vi "Create Channels.vi"(8 "error in (no error)":errorcluster, 10 "RSI Module in":refnum<class "9401.lvclass">, 11 "Parent Ref in":T1 format="%.0x") -> (0 "error out":errorcluster, 2 "RSI Module out":refnum<class "9401.lvclass">, 3 "Parent Ref out":T1 format="%.0x")   [LabVIEW 2017, in "Modules.lvlib" / "9401.lvclass"]
uses:
  9401.lvclass
  C:/Users/dbuck/Documents/GitHub/Scan-Engine-Custom-Device-Classes/Source/RSI Module/RSI Module.lvclass
  <vilib>/NI Veristand/Custom Device API/Custom Device Item Ref.ctl
  <vilib>/NI Veristand/Custom Device API/Custom Device Channel Type.ctl
  <vilib>/NI Veristand/Custom Device API/Custom Device Channel.ctl
  9401.lvclass/9401.ctl
  RSI Module/Class Property Strings.vi
  RSI Module/Channel GUIDs.vi
  <vilib>/NI Veristand/Custom Device API/Custom Device API.lvlib
  RSI Module/RSI Module.lvclass
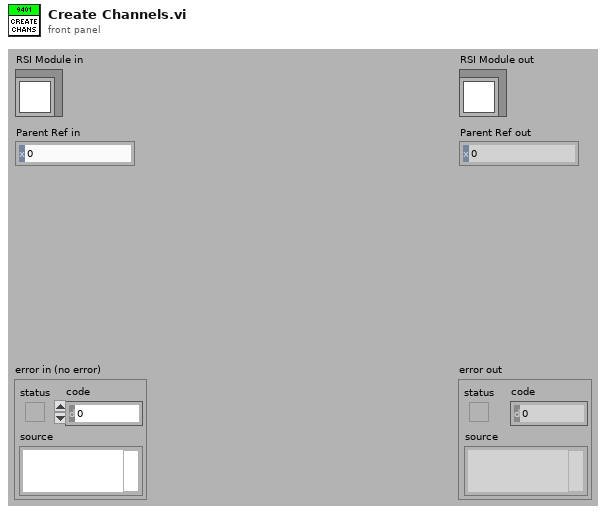
[diagram p1: front panel]
types:
  T1 = typedef "Custom Device API.lvlib/Custom Device Item Ref.ctl" = u64
  T2 = typedef "Custom Device API.lvlib/Custom Device Channel.ctl" = cluster{"Type":T3, "Units":string, "Default Value":dbl, "Faultable":bool, "Scalable":bool}
  T3 = typedef "Custom Device API.lvlib/Custom Device Channel Type.ctl" = enum16{"Input", "Output"}
  T4 = typedef "Modules.lvlib/RSI Module.lvclass/Channels.ctl" = cluster{"# Input Channels":i32, "# Output Channels":i32, "Channel Type":T5, "Units":string}
  T5 = typedef "Modules.lvlib/RSI Module.lvclass/Channel Type.ctl" = enum16{"Analog", "Digital"}
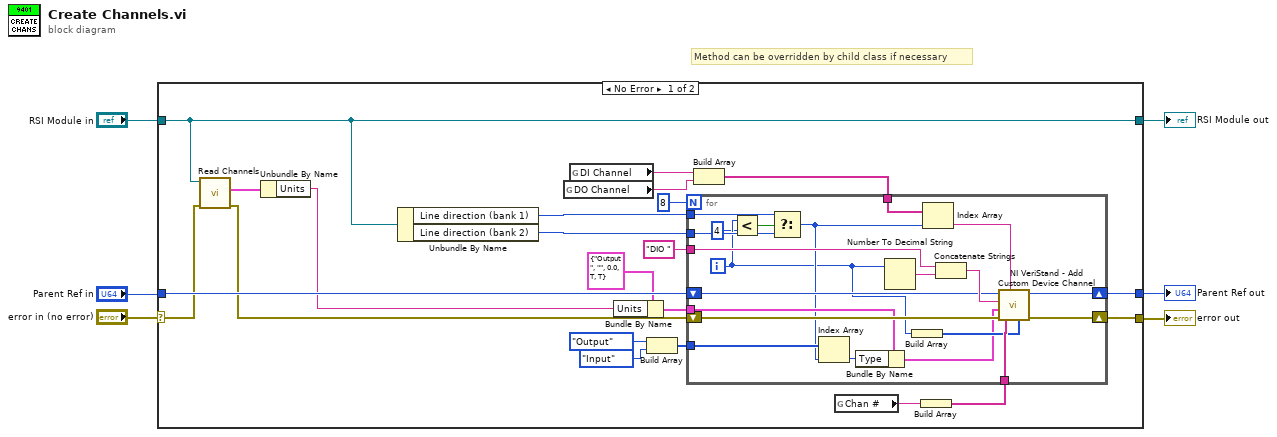
[diagram p0: block diagram]
diagram:
  # "Method can be overridden by child class if necessary"
  n1 = case shown="No Error" "error in (no error)" {
    selector: "error in (no error)" -> [w18 w52]
    tunnel: [w8 w52] -> w5
    tunnel: [w13 w51] -> w3
    tunnel: "RSI Module in" -> [w13 w51]
    tunnel: "Parent Ref in" -> [w23 w50]
    tunnel: [w9 w50] -> w1
    frame No Error {
      n2 = call "Read Channels.vi"("error in (no error)"=w18, "RSI Module in"=w13) -> ("error out"=w17:errorcluster, "Channels"=w19:T4)  [unwired: 7 in, 1 out]
      n3 = Unbundle By Name(w19) -> ("Units"=w20:string)
      n4 = Unbundle By Name(w13) -> ("Line direction (bank 1)"=w12:u32, "Line direction (bank 2)"=w7:u32)
      n5 = global read "Channel GUIDs.vi" "DO Channel"() -> (w27:string)
      n6 = global read "Channel GUIDs.vi" "DI Channel"() -> (w28:string)
      n7 = Bundle By Name(cluster=T2 {"Type"=enum."Output", "Units"="", "Default Value"=0.0, "Faultable"=TRUE, "Scalable"=TRUE} ("Channel"), "Units"=w20) -> (w14:T2)
      n8 = Build Array(Custom_Device_Channel_Type."Output" ("Type"), Custom_Device_Channel_Type."Input" ("Type")) -> (w11:T3[])
      n9 = Build Array(w28, w27) -> (w24:string[])
      n10 = global read "Class Property Strings.vi" "Chan #"() -> (w22:string)
      n11 = Build Array(w22) -> (w21:string[])
      n12 = for {
        N: 8 -> [_]
        tunnel: "DIO " ("Channel Name") -> [w47]
        tunnel: w14 -> [w38]
        tunnel: w24 -> [w40]
        tunnel: w21 -> [w44]
        shift-right: [w42] -> w8
        shift-left: w17 -> [w48]
        shift-right: [w41] -> w9
        shift-left: w23 -> [w45]
        tunnel: w12 -> [w34]
        tunnel: w11 -> [w37]
        tunnel: w7 -> [w32]
        i -> [w31]
        n13 = Less?(x=w31, y=4) -> (x < y?=w29:bool)
        n14 = Select(t=w34, s=w29, f=w32) -> (s? t:f=w33:u32)
        n15 = Index Array(array=w37, index=w33) -> (element=w36:T3)
        n16 = Bundle By Name(cluster=w38, "Type"=w36) -> (w35:T2)
        n17 = Number To Decimal String(number=w31) -> (decimal integer string=w49:string)  [unwired: 1 in]
        n18 = Build Array(w31) -> (w43:i32[])
        n19 = Index Array(array=w40, index=w33) -> (element=w39:string)
        n20 = Concatenate Strings(w47, w49) -> (w46:string)
        n21 = call <vilib>:"NI VeriStand - Add Custom Device Channel.vi"("Property Values"=w43, "Property names"=w44, "GUID (Default Channel)"=w39, "error in (no error)"=w48, "Channel"=w35, "Channel Name"=w46, "Parent Ref in"=w45) -> ("error out"=w42:errorcluster, "Parent Ref out"=w41:T1)  [unwired: 1 in, 2 out]
      }
    }
    frame Error {
    }
  }
  "error out" <- w5
  "RSI Module out" <- w3
  "Parent Ref out" <- w1
